vi "UNDTStringToCluster2(SubVI).vi"(7 "index":i32, 8 "error in":errorcluster, 9 "Header size":i32=56, 10 "Проверка CRC8":bool=TRUE, 11 "data_in":u8[](array[numeric]) format="%02x") -> (0 "error out":errorcluster, 2 "CRC8Good":bool=TRUE, 3 "UNDT_Cluster 3":T1 {"Gain Coeff" format="%#_6e"; "Reserve 1" format="%02x"; "Mux TX/RX" format="%02x"; "ScanDelay" format="%02x"; "PacketCounter" format="%08x"; "SamplingInterval" format="%#_6e"; "Lose Packet" format="%08x"; "EncodersParam2" format="%016x"; "EncodersParam1" format="%016x"; "CRC 8" format="%02x"; "N chanel" format="%02x"; "N tick" format="%02x"; "Ncycle" format="%04x"; "FrameFormatVersion" format="%02x"; "MagicWord" format="%.0x"}, 4 "SizeToSmall":bool)   [LabVIEW 2017]
uses:
  Control_EU/UNDT_ClusterPackRevers (Type).ctl
panel:
  out "length":i32
  out "x+y":i32
  out "CRC8_CCITT":u8=139 format="%1x"
  out "CRC8":u8=139 format="%02x"
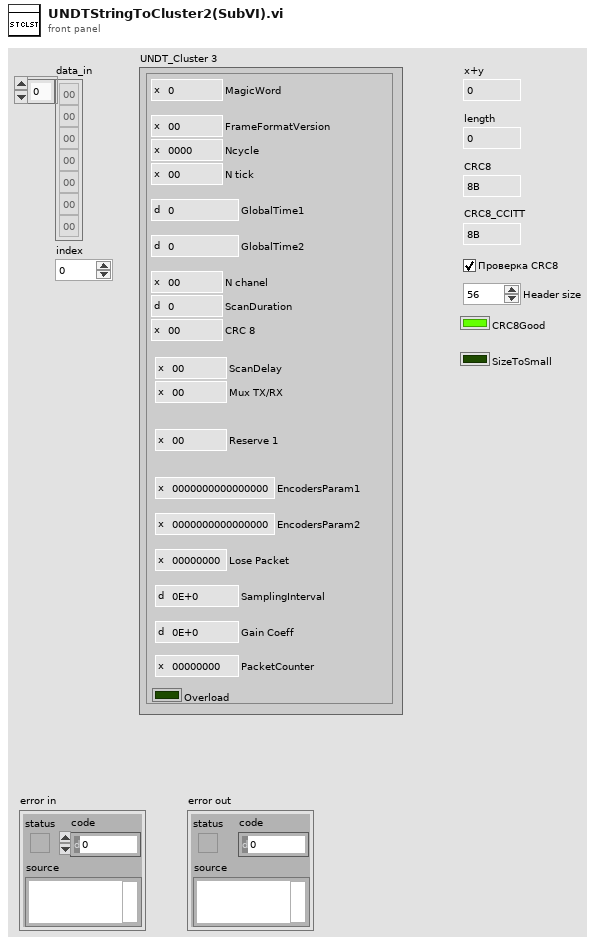
[diagram p1: front panel]
types:
  T1 = typedef "UNDT_ClusterPackRevers (Type).ctl" = cluster{"PacketCounter":u32, "Gain Coeff":sgl, "SamplingInterval":sgl, "Lose Packet":u32, "EncodersParam2":u64, "EncodersParam1":u64, "Reserve 1":u8, "Mux TX/RX":u8, "ScanDelay":u16, "CRC 8":u8, "ScanDuration":u16, "N chanel":u8, "GlobalTime2":u32, "GlobalTime1":u32, "N tick":u8, "Ncycle":u16, "FrameFormatVersion":u8, "MagicWord":u32, "Overload":bool}
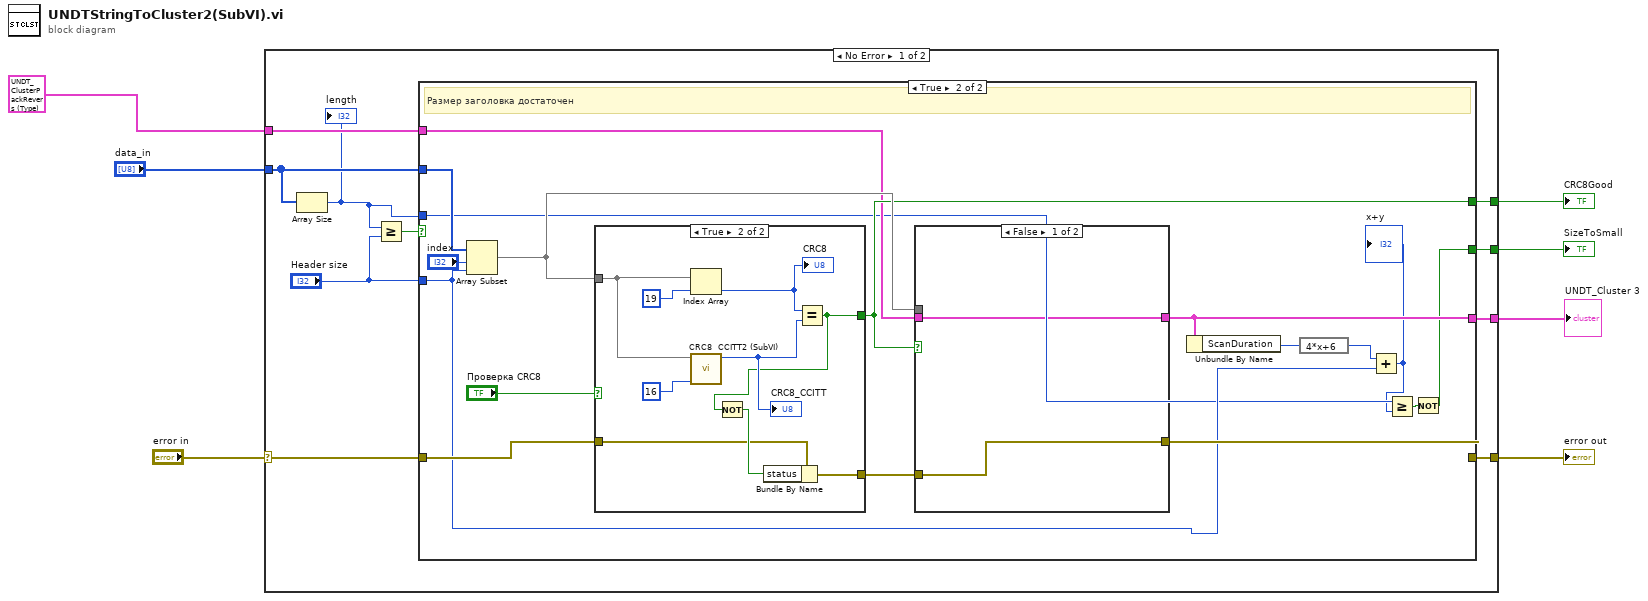
[diagram p0: block diagram]
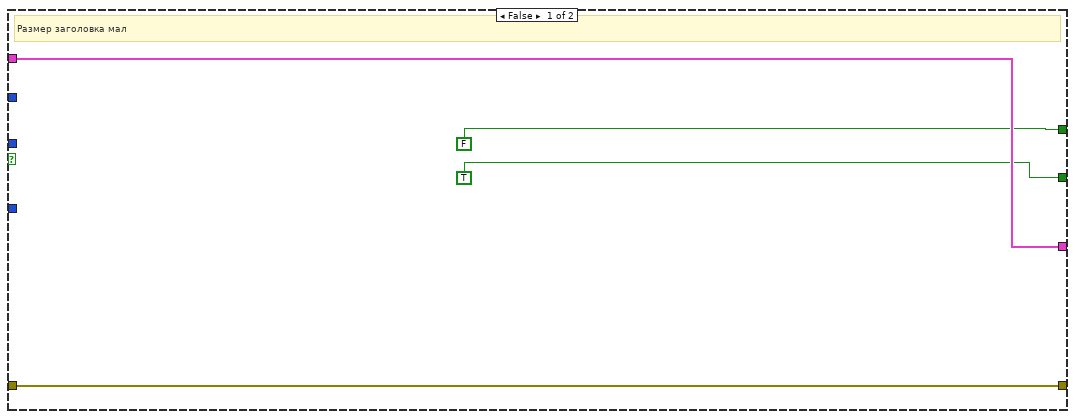
[diagram p2: hidden frame]
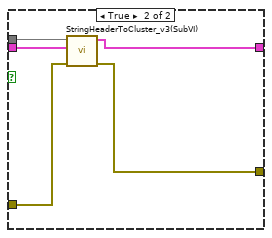
[diagram p3: hidden frame]
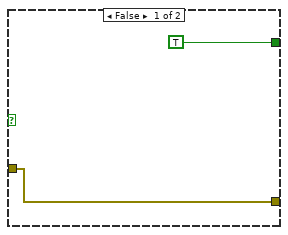
[diagram p4: hidden frame]
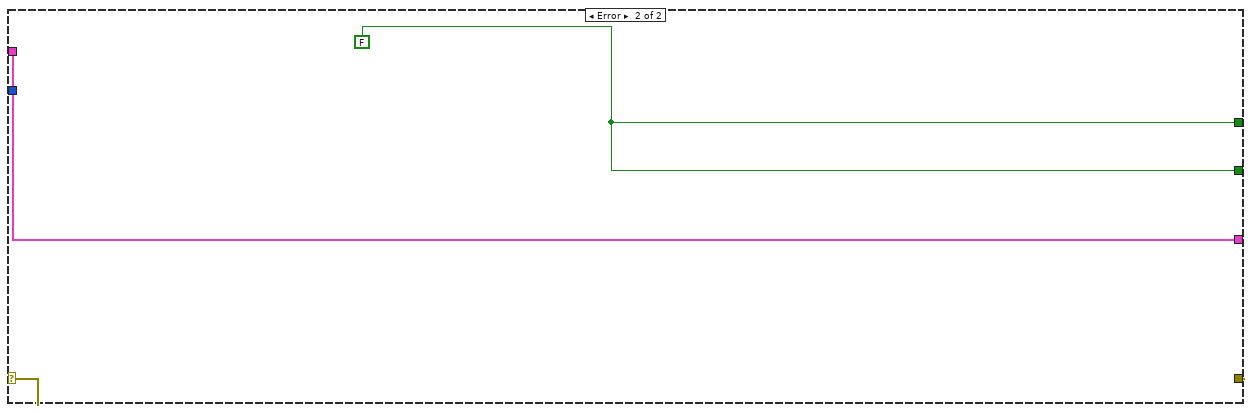
[diagram p5: hidden frame]
diagram:
  n1 = case shown="No Error" "error in" {
    selector: "error in" -> [w12 w58]
    tunnel: [w17 w57] -> w7
    tunnel: T1 {"PacketCounter"=0, "Gain Coeff"=0.0, "SamplingInterval"=0.0, "Lose Packet"=0, "EncodersParam2"=0, "EncodersParam1"=0, "Reserve 1"=0, "Mux TX/RX"=0, "ScanDelay"=0, "CRC 8"=0, "ScanDuration"=0, "N chanel"=0, "GlobalTime2"=0, "GlobalTime1"=0, "N tick"=0, "Ncycle"=0, "FrameFormatVersion"=0, "MagicWord"=0, "Overload"=FALSE} ("UNDT_Cluster 2") -> [w9 w59]
    tunnel: [w16 w59] -> w2
    tunnel: "data_in" -> [w15 _]
    tunnel: [w11 w58] -> w6
    tunnel: [w10 w57] -> w4
    frame No Error {
      n2 = Array Size(array=w15) -> (size(s)=w8:i32)
      "length" <- w8
      n3 = Greater Or Equal?(x=w8, y="Header size") -> (x >= y?=w13:bool)
      n4 = case shown="True" w13 {
        tunnel: [FALSE w36] -> w17
        tunnel: w9 -> [w21 w31]
        tunnel: [w21 w30] -> w16
        tunnel: w15 -> [_ w32]
        tunnel: "Header size" -> [_ w27]
        tunnel: w12 -> [w19 w35]
        tunnel: [w19 w34] -> w11
        tunnel: [TRUE w24] -> w10
        tunnel: w8 -> [_ w26]
        frame False {
          # "Размер заголовка мал"
        }
        frame True {
          # "Размер заголовка достаточен"
          n5 = Array Subset(array=w32, index="index", length=w27) -> (w37:u8[])
          n6 = case shown="True" "Проверка CRC8" {
            tunnel: w37 -> [_ w49]
            tunnel: [TRUE w53] -> w36
            tunnel: w35 -> [w46 w51]
            tunnel: [w46 w50] -> w33
            frame False {
            }
            frame True {
              n7 = Index Array(array=w49, index=19 ("offset (0)")) -> (element=w48:u8)
              "CRC8" <- w48
              n8 = call "CRC8  CCITT2 (SubVI).vi"("wLength"=16 ("length (rest)"), "unsigned byte array"=w49) -> ("CRC8_CCITT"=w54:u8)  [unwired: 9 in]
              "CRC8_CCITT" <- w54
              n9 = Equal?(x=w48, y=w54) -> (x = y?=w53:bool)
              n10 = Not(x=w53) -> (.not. x?=w52:bool)
              n11 = Bundle By Name(cluster=w51, "status"=w52) -> (w50:errorcluster)
            }
          }
          n12 = case shown="False" w36 {
            tunnel: w31 -> [w40 w42]
            tunnel: w37 -> [_ w45]
            tunnel: [w40 w41] -> w30
            tunnel: [w39 w43] -> w34
            tunnel: w33 -> [w39 w44]
            frame False {
            }
            frame True {
              n13 = call "StringHeaderToCluster_v3(SubVI).vi"("error in"=w44, "UNDT_Cluster 2"=w42, "data_in 2"=w45) -> ("error out"=w43:errorcluster, "UNDT_Cluster"=w41:T1)  [unwired: 7 in]
            }
          }
          n14 = Unbundle By Name(w30) -> ("ScanDuration"=w29:u16)
          n15 = expression code="4*x+6"(w29) -> (w28:u16)
          n16 = Add(x=w28, y=w27) -> (x+y=w25:i32)
          "x+y" <- w25
          n17 = Greater Or Equal?(x=w26, y=w25) -> (x >= y?=w23:bool)
          n18 = Not(x=w23) -> (.not. x?=w24:bool)
        }
      }
    }
    frame Error {
      w57 = FALSE
    }
  }
  "CRC8Good" <- w7
  "error out" <- w6
  "SizeToSmall" <- w4
  "UNDT_Cluster 3" <- w2
